vi "NF LI56xx sub init osc.vi"(8 "error in":errorcluster caption="error in (no error)" {"code" format="%.0x"}, 11 "VISA resource name":refnum<visa-resource-name>) -> (0 "error out":errorcluster {"code" format="%.0x"}, 3 "VISA resource name copy":refnum<visa-resource-name>)   [LabVIEW 2019]
doc: "get OSC related parameters"
panel:
  out "OSC output Cluster":T1
  in  "OSC Cluster":T1
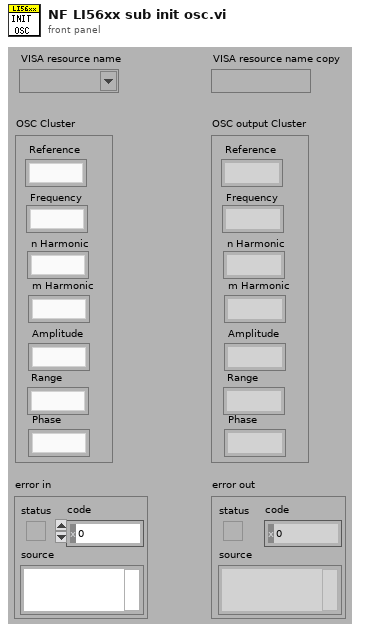
[diagram p1: front panel]
types:
  T1 = cluster{"Reference":string, "Frequency":string, "n Harmonic":string, "m Harmonic":string, "Amplitude":string, "Range":string, "Phase":string}
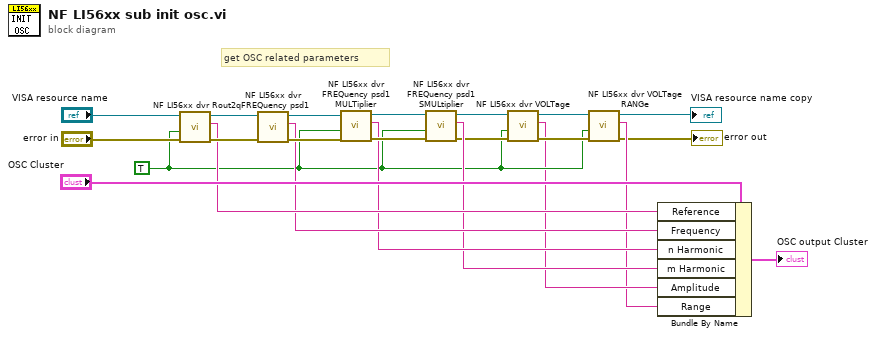
[diagram p0: block diagram]
diagram:
  w5 = TRUE ("Read(F)")
  # "get OSC related parameters"
  n1 = call "NF LI56xx dvr Rout2.vi"("error in"="error in", "Read(F)"=w5, "VISA resource name"="VISA resource name") -> ("error out"=w20:errorcluster, "query reference signal \nsource"=w14:string, "VISA resource name copy"=w21:refnum<visa-resource-name>)  [unwired: 6 in]
  n2 = call "NF LI56xx dvr qFREQuency psd1.vi"("error in"=w20, "VISA resource name"=w21) -> ("error out"=w18:errorcluster, "query Frequency"=w13:string, "VISA resource name copy"=w19:refnum<visa-resource-name>)  [unwired: 7 in]
  n3 = call "NF LI56xx dvr FREQuency psd1 MULTiplier.vi"("error in"=w18, "Read(F)"=w5, "VISA resource name"=w19) -> ("error out"=w16:errorcluster, "query harmonic order"=w12:string, "VISA resource name copy"=w17:refnum<visa-resource-name>)  [unwired: 6 in]
  n4 = call "NF LI56xx dvr FREQuency psd1 SMULtiplier.vi"("error in"=w16, "Read(F)"=w5, "VISA resource name"=w17) -> ("error out"=w8:errorcluster, "query subharmonic order"=w11:string, "VISA resource name copy"=w9:refnum<visa-resource-name>)  [unwired: 6 in]
  n5 = call "NF LI56xx dvr VOLTage.vi"("error in"=w8, "Read(F)"=w5, "VISA resource name"=w9) -> ("error out"=w7:errorcluster, "query AC Voltage"=w4:string, "VISA resource name copy"=w6:refnum<visa-resource-name>)  [unwired: 6 in]
  n6 = call "NF LI56xx dvr VOLTage RANGe.vi"("error in"=w7, "Read(F)"=w5, "VISA resource name"=w6) -> ("error out"=→"error out":errorcluster, "query AC Voltage"=w3:string, "VISA resource name copy"=→"VISA resource name copy":refnum<visa-resource-name>)  [unwired: 6 in]
  n7 = Bundle By Name(cluster="OSC Cluster", "Reference"=w14, "Frequency"=w13, "n Harmonic"=w12, "m Harmonic"=w11, "Amplitude"=w4, "Range"=w3) -> (→"OSC output Cluster":T1)
